vi "Verify_ACK.vi"(4 "error code":i32, 5 "error code description":string="error code description", 6 "error in (no error)":errorcluster, 9 "connection ID":refnum<k5>) -> (0 "error out":errorcluster, 3 "connection ID out":refnum<k5>)   [LabVIEW 2025, in "CAENels FAST-PS.lvlib"]
uses:
  CAENels FAST-PS.lvlib
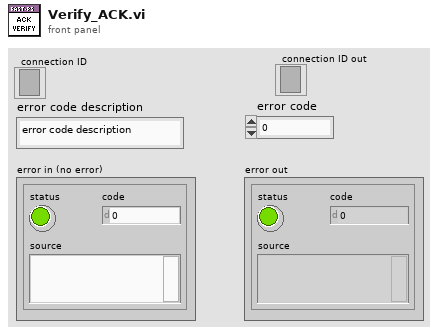
[diagram p1: front panel]
types:
  T1 = enum16{"Standard", "Buffered", "CRLF", "Immediate"}
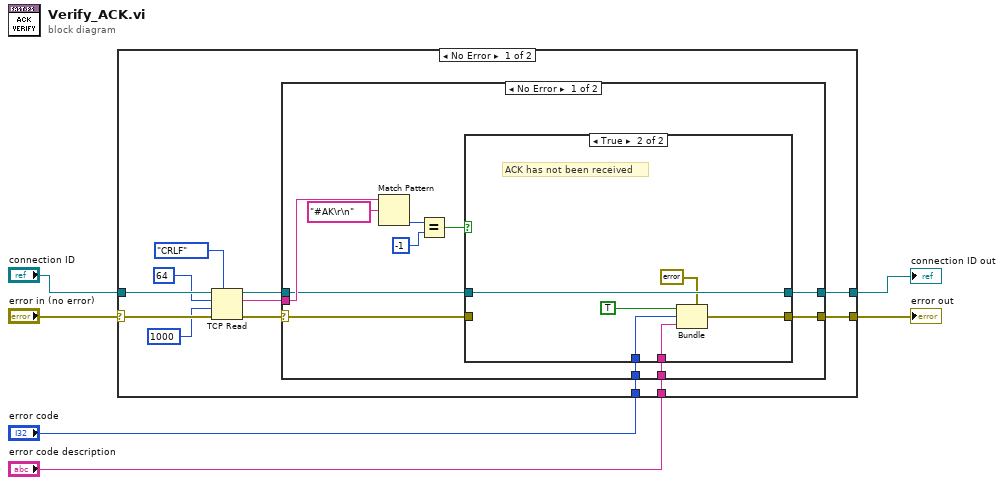
[diagram p0: block diagram]
diagram:
  n1 = case shown="No Error" "error in (no error)" {
    selector: "error in (no error)" -> [w18 w41]
    tunnel: "connection ID" -> [w17 w40]
    tunnel: [w12 w41] -> w4
    tunnel: [w11 w40] -> w3
    tunnel: "error code" -> [w8 _]
    tunnel: "error code description" -> [w7 _]
    frame No Error {
      n2 = TCP Read(connection ID=w17, bytes to read=64, error in (no error)=w18, 7:T1."CRLF" ("mode (standard)"), 9:1000 ("timeout ms (25000)")) -> (connection ID out=w10:refnum<k5>, data out=w9:string, error out=w13:errorcluster)
      n3 = case shown="No Error" w13 {
        selector: w13 -> [w24 w39]
        tunnel: [w23 w39] -> w12
        tunnel: [w21 w38] -> w11
        tunnel: w10 -> [w22 w38]
        tunnel: w9 -> [w28 _]
        tunnel: w8 -> [w20 _]
        tunnel: w7 -> [w19 _]
        frame No Error {
          n4 = Match Pattern(string=w28, regular expression="#AK\r\n") -> (offset past match=w27:i32)  [unwired: 4 out]
          n5 = Equal?(x=w27, y=-1) -> (x = y?=w25:bool)
          n6 = case shown="True" w25 {
            tunnel: [w31 w36] -> w23
            tunnel: w24 -> [w31 _]
            tunnel: w22 -> [w30 w37]
            tunnel: [w30 w37] -> w21
            tunnel: w20 -> [_ w33]
            tunnel: w19 -> [_ w32]
            frame False {
              # "ACK has been found"
            }
            frame True {
              # "ACK has not been received"
              n7 = Bundle(cluster=errorcluster {"status"=FALSE, "code"=0, "source"=""} ("error in  2"), "status"=TRUE, "code"=w33, "source"=w32) -> (w36:errorcluster)
            }
          }
        }
        frame Error {
        }
      }
    }
    frame Error {
    }
  }
  "error out" <- w4
  "connection ID out" <- w3
